vi "FG - StatusStrRef.vi"(0 "StatusStr Ref in":refnum<vi>, 1 "error in (no error)":errorcluster, 4 "action (Get)":T1=enum."Get") -> (7 "StatusStr Ref out":refnum<vi>, 8 "error out":errorcluster)   [LabVIEW 2020]
doc: "Developed by Kevin Thompson\nkevin@thompsonengineering.net\n\nCopyright 2018-2020\nThompson Engineering, LLC"
uses:
  DataTypes/TD GetSet ActionSelect--enum.ctl
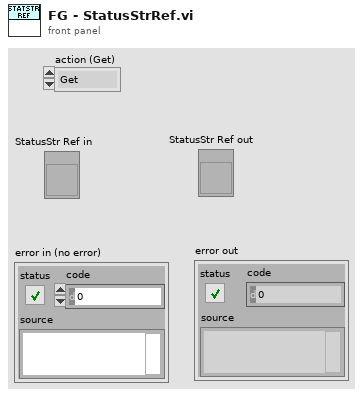
[diagram p1: front panel]
types:
  T1 = typedef "TD GetSet ActionSelect--enum.ctl" = enum16{"Init", "Get", "Set"}
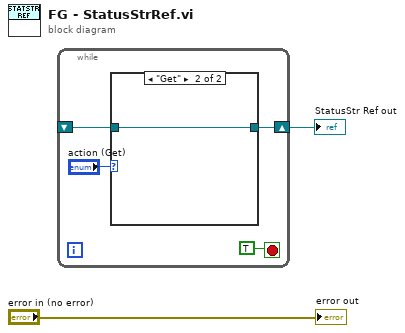
[diagram p0: block diagram]
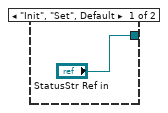
[diagram p2: hidden frame]
diagram:
  n1 = while {
    shift-right: [w3] -> w1
    shift-left: _ -> [w4]
    stop <- TRUE stop-if-true
    n2 = case shown="\"Get\"" "action (Get)" {
      tunnel: w4 -> [_ w8]
      tunnel: ["StatusStr Ref in" w8] -> w3
      frame "Init", "Set", Default {
      }
      frame "Get" {
      }
    }
  }
  "StatusStr Ref out" <- w1
  "error out" <- "error in (no error)"
